vi "Format File Path for Linux.vi"(8 "error in (no error)":errorcluster, 11 "Path":string) -> (0 "error out":errorcluster, 3 "Path out":string)   [LabVIEW 2015, in "Waveform Data Logger Shared.lvlib"]
uses:
  Waveform Data Logger Shared.lvlib
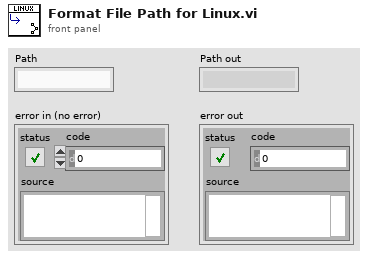
[diagram p1: front panel]
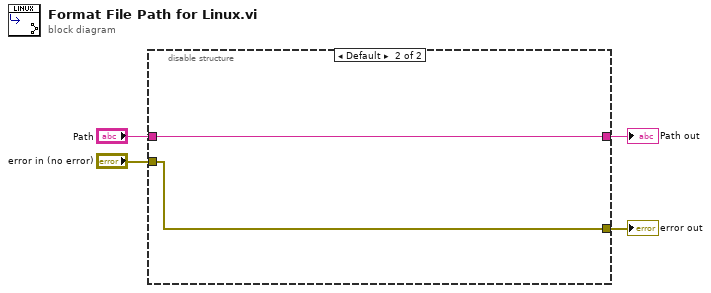
[diagram p0: block diagram]
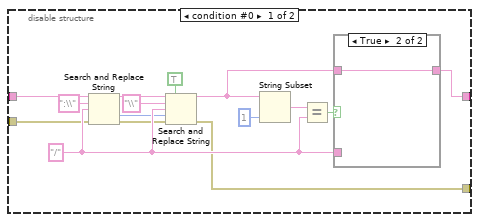
[diagram p2: hidden frame]
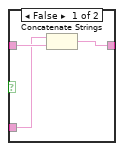
[diagram p3: hidden frame]
diagram:
  n1 = disable-structure shown="Default" {
    disable-tunnel: "Path" -> [w18 w25]
    disable-tunnel: [w9 w25] -> w2
    disable-tunnel: "error in (no error)" -> [w6 w24]
    disable-tunnel: [w5 w24] -> w4
    frame condition #0 {
      w10 = "/" ("replace string (\"\")")
      n2 = Search and Replace String(input string=w18, search string=":\\", replace string=w10, error in=w6) -> (result string=w17:string, offset past replacement=w7:i32, error out=w8:errorcluster)  [unwired: 4 in, 1 out]
      n3 = Search and Replace String(replace all?=TRUE ("replace all? (F)"), input string=w17, search string="\\", replace string=w10, offset=w7, error in=w8) -> (result string=w11:string, error out=w5:errorcluster)  [unwired: 2 in, 2 out]
      n4 = String Subset(string=w11, length (rest)=1 ("length (rest)")) -> (substring=w13:string)  [unwired: 1 in]
      n5 = Equal?(x=w13, y=w10) -> (x = y?=w12:bool)
      n6 = case shown="True" w12 {
        tunnel: w11 -> [w22 w23]
        tunnel: w10 -> [w21 _]
        tunnel: [w20 w23] -> w9
        frame False {
          n7 = Concatenate Strings(w21, w22) -> (w20:string)
        }
        frame True {
        }
      }
    }
    frame condition #1 (active) {
    }
  }
  "error out" <- w4
  "Path out" <- w2
